vi "Grid_Calibration.vi"() -> ()   [LabVIEW 2017]
panel:
  out "error out":errorcluster
  out "Corrected Image":T1(plugin-control)
  out "Original Image":T1(plugin-control)
  in  "File Path":path
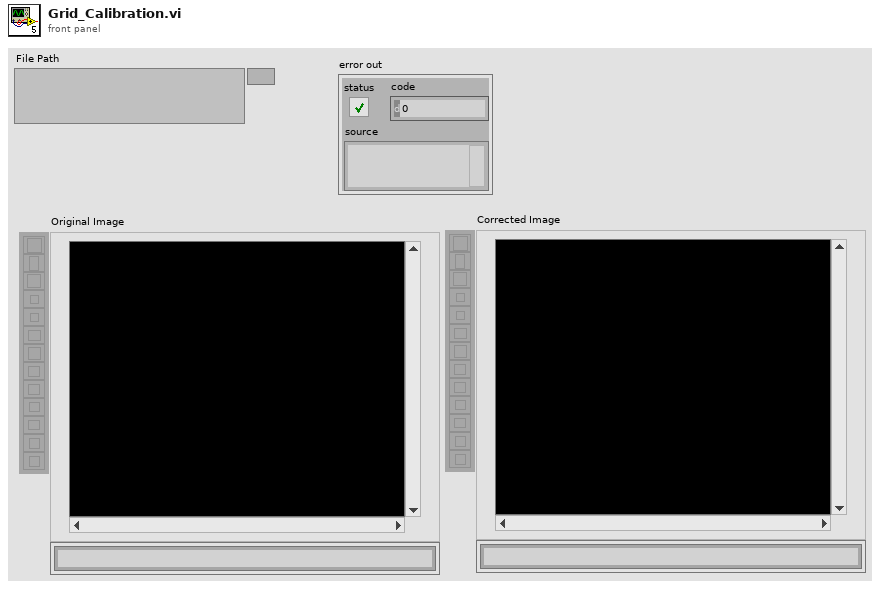
[diagram p1: front panel]
types:
  T1 = typedef "IMAQ Image.ctl" = refnum<image>
  T2 = typedef "Image Type" = u32
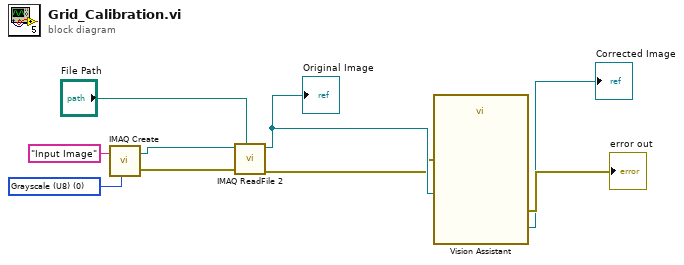
[diagram p0: block diagram]
diagram:
  w8 = T2 0 items=["Grayscale (U8)", "Grayscale (I16)", "Grayscale (SGL)", "Complex (CSG)", "RGB (U32)", "HSL (U32)", "RGB (U64)", "Grayscale (U16)"] ("Image Type")
  n1 = call "IMAQ Create"("Image Name"="Input Image", "Image Type"=w8) -> ("New Image"=w7:T1, "error out"=w6:errorcluster)  [unwired: 3 in]
  n2 = call "IMAQ ReadFile 2"("File Path"="File Path", "error in (no error)"=w6, "Image"=w7) -> ("error out"=w3:errorcluster, "Image Out"=w4:T1)  [unwired: 4 in, 3 out]
  "Original Image" <- w4
  n3 = call "Vision Assistant"("Image In"=w4, "error in"=w3) -> ("Image Out"=→"Corrected Image":T1, "error out"=→"error out":errorcluster)  [unwired: 24 in]
